vi "Protocol.Command.Convert Internal Command.vi"(8 "error in (no error)":errorcluster, 11 "Value":dbl) -> (0 "error out":errorcluster, 3 "Enum":T1)   [LabVIEW 2023, in "J1939 Addon Engine.lvlib"]
uses:
  J1939 Addon Engine.lvlib
  Types/Protocol.Command.States.ctl
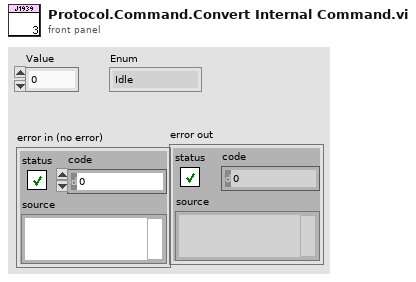
[diagram p1: front panel]
types:
  T1 = typedef "J1939 Addon Engine.lvlib/Protocol.Command.States.ctl" = enum8{"Idle", "Refresh Address", "Verify DTCs", "Clear DTCs", "Clear Status Bit", "Clear Error Bit"}
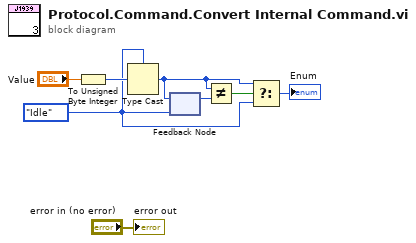
[diagram p0: block diagram]
diagram:
  w1 = Protocol.Command.States."Idle"
  n1 = To Unsigned Byte Integer(number="Value") -> (unsigned 8bit integer=w3:u8)
  n2 = Type Cast(type=w1, x=w3) -> (*(type *) &x=w6:T1)
  n3 = feedback #1(w1) -> (w4:T1)
  n4 = feedback-in #1(w6) -> ()
  n5 = Not Equal?(x=w6, y=w4) -> (x != y?=w5:bool)
  n6 = Select(t=w6, s=w5, f=w1) -> (s? t:f=→"Enum":T1)
  "error out" <- "error in (no error)"
